vi "subSave_DaqInfo.vi"(8 "full path":path, 11 "Waveform info":T1={"Waveform folder"=path "C:/Users/ZouOptics/Desktop/MATLAB codes/ephys waveforms_new/triangle -100 to 50", "Movie frame rate (Hz)"=1000.0} {"Movie frame rate (Hz)" format="%0.0f"}) -> ()   [LabVIEW 2015]
panel:
  # "This VI copies the waveform data folder to the DAQ data file folder"
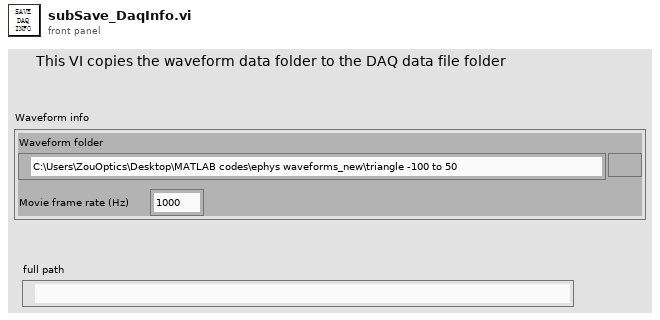
[diagram p1: front panel]
types:
  T1 = cluster{"Waveform folder":path, "Movie frame rate (Hz)":dbl}
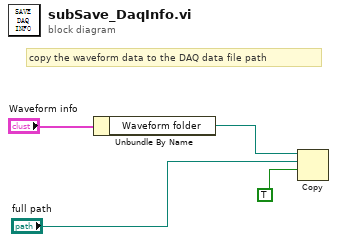
[diagram p0: block diagram]
diagram:
  # "copy the waveform data to the DAQ data file path"
  n1 = Unbundle By Name("Waveform info") -> ("Waveform folder"=w3:path)
  n2 = Copy(9:TRUE ("overwrite (F)"), 10:"full path", 11:w3) -> ()  [unwired: 2 in, 3 out]
